vi "Get_Next_Sub_Collection.vi"(8 "error in (no error)":errorcluster caption="entrée d'erreur (pas d'erreur)", 11 "Firebase AssembledProducts en entrée":refnum<class "Firebase AssembledProducts_Booleen.lvclass">) -> (0 "error out":errorcluster caption="sortie d'erreur", 3 "Firebase AssembledProducts en sortie":refnum<class "Firebase AssembledProducts_Booleen.lvclass">)   [LabVIEW 2020, in "Library Instrument & Equipement.lvlib" / "Library FireBase.lvlib" / "Firebase AssembledProducts_Booleen.lvclass"]
doc: "Return the documents present in the test collection for each DATA read with Get_Data\nPlease initialise the following values\n - Name BDD\n - Document of test sequence\n - API Key\n - Nb To Read"
uses:
  Firebase AssembledProducts_Booleen.lvclass
  C:/Users/ngarcin/OneDrive - Altyor/Standard TB/Class/Firebase/Source/Firebase AssembledProducts/Firebase AssembledProducts.lvclass
  C:/Users/ngarcin/OneDrive - Altyor/Standard TB/Class/Firebase/Source/Firebase Driver/Firebase Driver.lvclass
  Firebase AssembledProducts_Booleen.lvclass/Firebase AssembledProducts_Booleen.ctl
  JSON API/JSON Value/JSON Value.lvclass
  JSON API/JSON Value/Set from JSON string.vi
  Firebase AssembledProducts.lvclass
  JSON API/Variant JSON/Variant JSON.lvlib
  JSON API/Get Polymorphic/JSON GetSet.lvlib
  Firebase Driver/Firebase Driver.lvclass
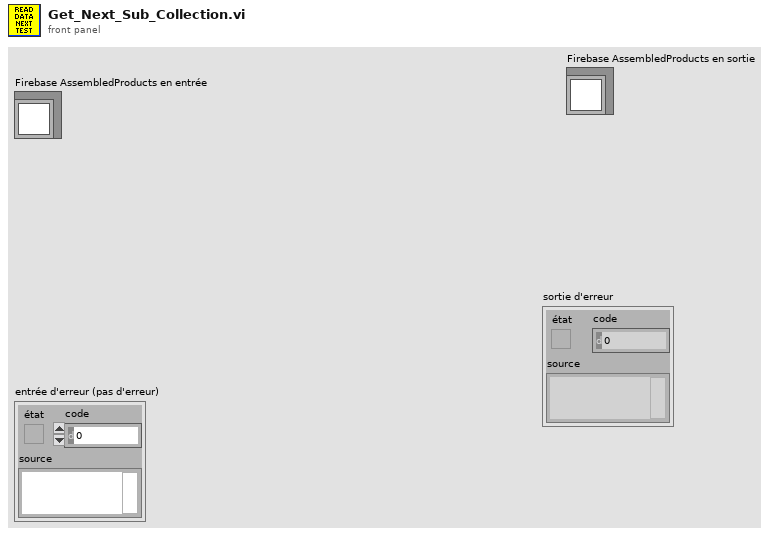
[diagram p1: front panel]
types:
  T1 = cluster{"name":string, "fields":cluster{"Result":cluster{"booleanValue":bool}, "Name":cluster{"stringValue":string}, "StartOfTest":cluster{"timestampValue":string}, "EndOfTest":cluster{"timestampValue":string}, "limit":cluster{"mapValue":cluster{"fields":cluster{"Lower":cluster{"stringValue":string}, "Upper":cluster{"stringValue":string}}}}, "Value":cluster{"booleanValue":bool}, "Type":cluster{"stringValue":string}, "MainTest":cluster{"stringValue":string}}}[][]
  T2 = cluster{"name":string, "fields":cluster{"Result":cluster{"booleanValue":bool}, "CreationDate":cluster{"timestampValue":string}, "Batch":cluster{"stringValue":string}, "SerialNumber":cluster{"stringValue":string}, "EndOfProduction":cluster{"timestampValue":string}, "FW_Version":cluster{"mapValue":cluster{"fields":cluster{"Bootloader":cluster{"mapValue":cluster{"fields":cluster{"File_Name":cluster{"stringValue":string}, "Version":cluster{"mapValue":cluster{"fields":cluster{"Major":cluster{"stringValue":string}, "Minor":cluster{"stringValue":string}}}}, "Checksum":cluster{"stringValue":string}}}}, "SoftDevice":cluster{"mapValue":cluster{"fields":cluster{"File_Name":cluster{"stringValue":string}, "Version":cluster{"mapValue":cluster{"fields":cluster{"Major":cluster{"stringValue":string}, "Minor":cluster{"stringValue":string}}}}, "Checksum":cluster{"stringValue":string}}}}, "DFU":cluster{"mapValue":cluster{"fields":cluster{"File_Name":cluster{"stringValue":string}, "Version":cluster{"mapValue":cluster{"fields":cluster{"Major":cluster{"stringValue":string}, "Minor":cluster{"stringValue":string}}}}, "Checksum":cluster{"stringValue":string}}}}}}}, "PartNumber":cluster{"stringValue":string}, "OrderNumber":cluster{"stringValue":string}, "Operator":cluster{"stringValue":string}, "AssembledProductName":cluster{"stringValue":string}}}[]
  T3 = cluster{"name":string, "fields":cluster{"Result":cluster{"booleanValue":bool}, "Name":cluster{"stringValue":string}, "StartOfTest":cluster{"timestampValue":string}, "EndOfTest":cluster{"timestampValue":string}, "limit":cluster{"mapValue":cluster{"fields":cluster{"Lower":cluster{"stringValue":string}, "Upper":cluster{"stringValue":string}}}}, "Value":cluster{"booleanValue":bool}, "Type":cluster{"stringValue":string}, "MainTest":cluster{"stringValue":string}}}[]
  T4 = cluster{"documents":cluster{"name":string, "fields":cluster{"Result":cluster{"booleanValue":bool}, "Name":cluster{"stringValue":string}, "StartOfTest":cluster{"timestampValue":string}, "EndOfTest":cluster{"timestampValue":string}, "limit":cluster{"mapValue":cluster{"fields":cluster{"Lower":cluster{"stringValue":string}, "Upper":cluster{"stringValue":string}}}}, "Value":cluster{"booleanValue":bool}, "Type":cluster{"stringValue":string}, "MainTest":cluster{"stringValue":string}}}[], "nextPageToken":string}
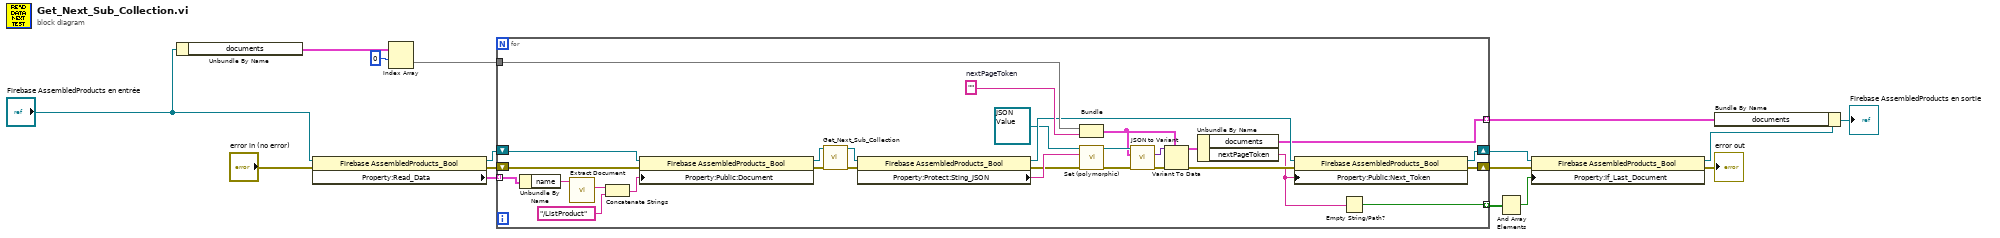
[diagram p0: block diagram]
diagram:
  n1 = Unbundle By Name("Firebase AssembledProducts en entrée") -> ("documents"=w16:T1)
  n2 = property class="Firebase AssembledProducts_Bool"(reference="Firebase AssembledProducts en entrée", error in="error in (no error)") -> (reference out=w11:refnum<class "Firebase AssembledProducts_Booleen.lvclass">, error out=w10:errorcluster, "Property:Read_Data"=w12:T2)
  n3 = Index Array(array=w16, index (row)=0 ("indice (ligne)")) -> (element=w15:T3)  [unwired: 1 in]
  n4 = for {
    tunnel: [w24] -> w1 mode=indexing
    shift-right: [w26] -> w8
    shift-left: w11 -> [w38]
    shift-right: [w28] -> w9
    shift-left: w10 -> [w37]
    tunnel: w12 -> [w36] mode=indexing
    tunnel: w15 -> [w31]
    tunnel: [w17] -> w13 mode=indexing
    w40 = ""  # nextPageToken
    n5 = Unbundle By Name(w36) -> ("name"=w35:string)
    n6 = call "Extract Document.vi"("Name"=w35) -> ("Source"=w34:string)  [unwired: 9 in, 1 out]
    n7 = Concatenate Strings(w34, "/ListProduct" ("chaîne")) -> (w32:string)
    n8 = property class="Firebase AssembledProducts_Bool"(reference=w38, error in=w37, "Property:Public:Document"=w32) -> (reference out=w19:refnum<class "Firebase AssembledProducts_Booleen.lvclass">, error out=w22:errorcluster)
    n9 = call-parent "Get_Next_Sub_Collection.vi"("error in (no error)"=w22, "Firebase AssembledProducts en entrée"=w19) -> ("error out"=w21:errorcluster, "Firebase AssembledProducts en sortie"=w20:refnum<class "Firebase AssembledProducts_Booleen.lvclass">)  [unwired: 8 in]
    n10 = property class="Firebase AssembledProducts_Bool"(reference=w20, error in=w21) -> (reference out=w27:refnum<class "Firebase AssembledProducts_Booleen.lvclass">, error out=w30:errorcluster, "Property:Protect:Sting_JSON"=w42:string)
    n11 = Bundle("documents"=w31, "nextPageToken"=w40) -> (w39:T4)  [unwired: 1 in]
    n12 = call-poly "Set (polymorphic).vi"("error in (no error)"=w30, "JSON stream"=w42, "JSON Value in"=refnum<class "JSON Value.lvclass"> refnum) -> ("error out"=w43:errorcluster, "JSON Value out"=w45:refnum<class "JSON Value.lvclass">)  [unwired: 6 in, 1 out]
    n13 = call "JSON to Variant.vi"("error in (no error)"=w43, "Variant (Data Type)"=w39, "JSON Value"=w45) -> ("error out"=w44:errorcluster, "Variant out"=w23:variant)  [unwired: 7 in]
    n14 = Variant To Data(error in=w44, type=w39, Variant=w23) -> (data=w41:T4, error out=w29:errorcluster)
    n15 = Unbundle By Name(w41) -> ("documents"=w24:T3, "nextPageToken"=w18:string)
    n16 = property class="Firebase AssembledProducts_Bool"(reference=w27, error in=w29, "Property:Public:Next_Token"=w18) -> (reference out=w26:refnum<class "Firebase AssembledProducts_Booleen.lvclass">, error out=w28:errorcluster)
    n17 = Empty String/Path?(string/path=w18) -> (empty?=w17:bool)
  }
  n18 = And Array Elements(Boolean array=w13) -> (logical AND=w6:bool)
  n19 = property class="Firebase AssembledProducts_Bool"(reference=w8, error in=w9, "Property:If_Last_Document"=w6) -> (reference out=w7:refnum<class "Firebase AssembledProducts_Booleen.lvclass">, error out=→"error out":errorcluster)
  n20 = Bundle By Name(cluster=w7, "documents"=w1) -> (→"Firebase AssembledProducts en sortie":refnum<class "Firebase AssembledProducts_Booleen.lvclass">)
